vi "Write Conversion Time.vi"(8 "error in":errorcluster, 10 "conversion time":T1, 11 "AI with conversion filter channel in":refnum<class "AI with Conversion Filter Channel.lvclass">) -> (0 "error out":errorcluster, 3 "AI with conversion filter channel out":refnum<class "AI with Conversion Filter Channel.lvclass">)   [LabVIEW 2017, in "Scan Engine Scripting.lvlib" / "AI with Conversion Filter Channel.lvclass"]
uses:
  AI with Conversion Filter Channel.lvclass
  Conversion Time.ctl
  AI with Conversion Filter Channel.lvclass/AI with Conversion Filter Channel.ctl
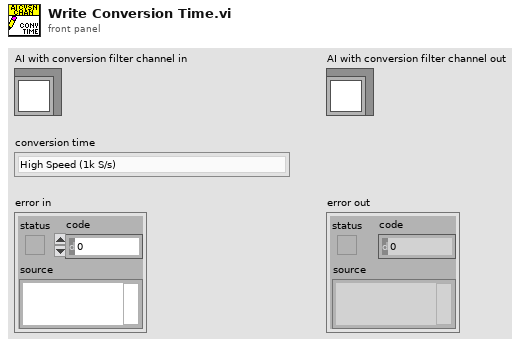
[diagram p1: front panel]
types:
  T1 = typedef "Scan Engine Scripting.lvlib/AI with Conversion Filter Channel.lvclass/Conversion Time.ctl" = enum16{"High Speed (1k S/s)", "Medium Speed (100 S/s)", "Medium Resolution (50/60 Hz Rejection - 12 S/s)", "High Resolution (50/60 Hz Rejection - 2 S/s)"}
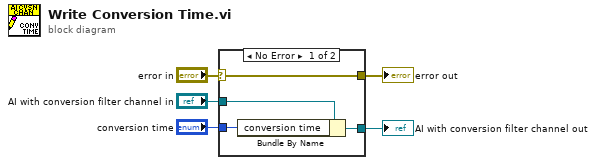
[diagram p0: block diagram]
diagram:
  n1 = case shown="No Error" "error in" {
    selector: "error in" -> [w9 w10]
    tunnel: [w9 w10] -> w4
    tunnel: [w7 w11] -> w2
    tunnel: "AI with conversion filter channel in" -> [w8 w11]
    tunnel: "conversion time" -> [w6 _]
    frame No Error {
      n2 = Bundle By Name(cluster=w8, "conversion time"=w6) -> (w7:refnum<class "AI with Conversion Filter Channel.lvclass">)
    }
    frame Error {
    }
  }
  "error out" <- w4
  "AI with conversion filter channel out" <- w2
